vi "loadXYpositions.vi"() -> ()   [LabVIEW 2013]
uses:
  <vilib>/Analysis/Matrix/Datatypes/RealMatrix.ctl
  <vilib>/Analysis/Matrix/NI_Matrix.lvlib
panel:
  out "Number of lines":u32
  in  "Chemin 2":path
  out "final XY":T1
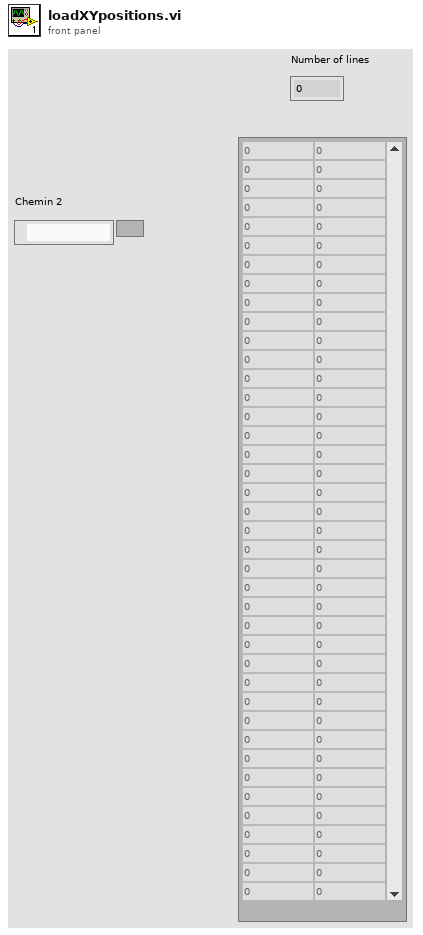
[diagram p1: front panel]
types:
  T1 = typedef "NI_Matrix.lvlib/RealMatrix.ctl" = dbl[][]
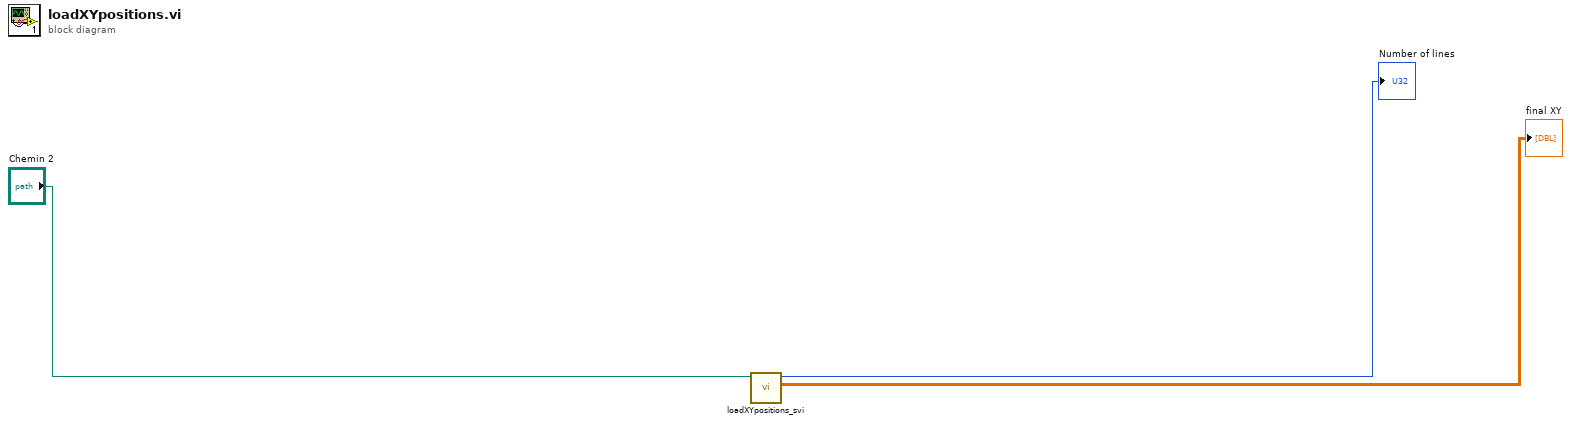
[diagram p0: block diagram]
diagram:
  n1 = call "loadXYpositions_svi.vi"("Chemin en entrée"="Chemin 2") -> ("final XY"=→"final XY":T1, "Number of lines"=→"Number of lines":u32)  [unwired: 9 in]
